vi "GetModuleName.vi"(5 "package":path, 9 "path in":path) -> (3 "path out":path, 4 "module":string)   [LabVIEW 2014, in "Python Functions.lvlib"]
uses:
  Python Functions.lvlib
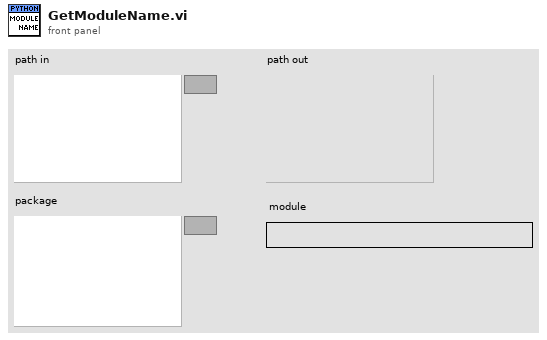
[diagram p1: front panel]
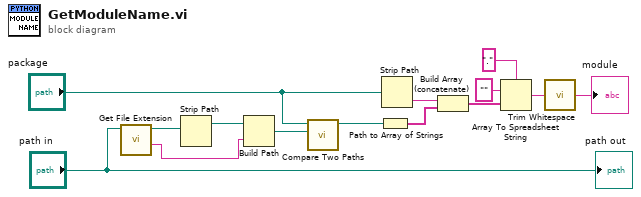
[diagram p0: block diagram]
diagram:
  n1 = call <vilib>:"Get File Extension.vi"("file"="path in") -> ("filename without extension"=w2:string, "dup file"=w4:path)  [unwired: 7 in, 2 out]
  n2 = Strip Path(path=w4) -> (stripped path=w3:path)  [unwired: 1 out]
  n3 = Build Path(base path=w3, name or relative path=w2) -> (appended path=w1:path)
  n4 = call <vilib>:"Compare Two Paths.vi"("Path 2"=w1, "Path 1"="package") -> ("Relative Path from 1 to 2"=w14:path)  [unwired: 6 in, 3 out]
  n5 = Path to Array of Strings(0:w14) -> (2:w11:string[])  [unwired: 1 out]
  n6 = Strip Path(path="package") -> (name=w12:string)  [unwired: 1 out]
  n7 = Build Array (concatenate)(w12, w11) -> (w10:string[])
  n8 = Array To Spreadsheet String(delimiter (Tab)=".", array=w10, 3:"" ("format string")) -> (spreadsheet string=w7:string)
  n9 = call <vilib>:"Trim Whitespace.vi"("string"=w7) -> ("trimmed string"=→"module":string)  [unwired: 1 in]
  "path out" <- "path in"
